vi "Get Transfer.vi"(10 "id":string, 11 "DSF Configuration in":T3) -> (0 "exists?":bool, 2 "info":T1, 3 "DSF Configuration out":T3, 4 "index":i32)   [LabVIEW 2017, in "DSF Core.lvlib" / "Configuration Session.lvclass"]
uses:
  Configuration Session.lvclass
  DSF Config Data.ctl
  Typedefs/DSF Timing Info.ctl
  DSF Core.lvlib
  Typedefs/DSF Version Info.ctl
  Internal DSF Configuration.ctl
  Typedefs/DSF Transfer Info.ctl
  Typedefs/DSF Byte Order.ctl
  Typedefs/DSF Settings Info.ctl
  Typedefs/DSF Engine Plugin Thread Configuration.ctl
  Typedefs/DSF File Format 1.0 Channel.ctl
  Typedefs/DSF File Format 1.0 Transfer.ctl
  Typedefs/DSF File Format 1.0 Transfer Group.ctl
  Typedefs/DSF File Format 1.0 Plugin.ctl
  Typedefs/DSF File Format 1.0 Framework v1.ctl
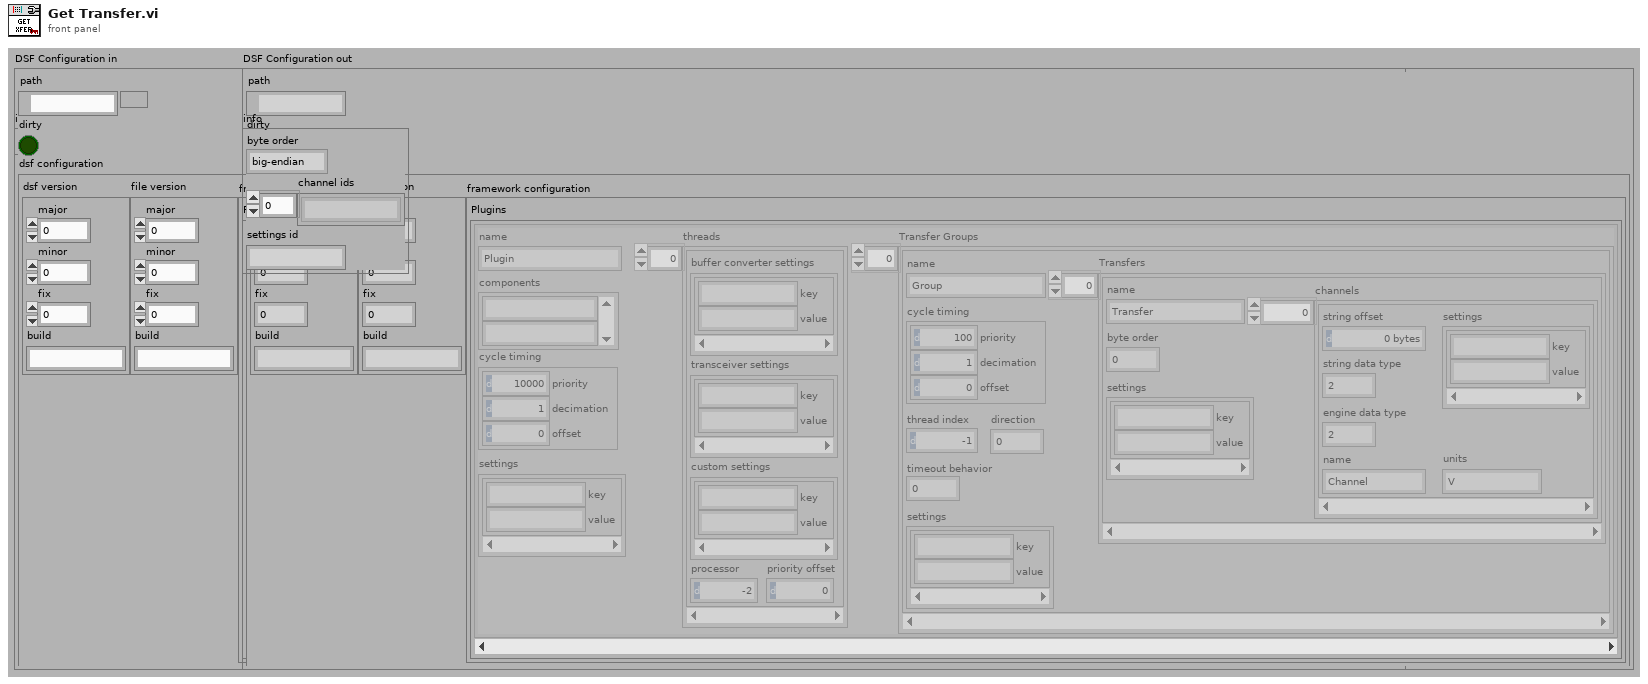
[diagram p1: front panel]
types:
  T1 = typedef "DSF Core.lvlib/DSF Transfer Info.ctl" = cluster{"byte order":T2, "channel ids":string[], "settings id":string}
  T2 = typedef "DSF Core.lvlib/DSF Byte Order.ctl" = enum8{"big-endian", "little-endian"}
  T3 = typedef "DSF Core.lvlib/Configuration Session.lvclass/DSF Config Data.ctl" = cluster{"path":path, "dirty":bool, "dsf configuration":T4}
  T4 = typedef "DSF Core.lvlib/Configuration Session.lvclass/Internal DSF Configuration.ctl" = cluster{"dsf version":T5, "file version":T5, "framework configuration":T6}
  T5 = typedef "DSF Core.lvlib/DSF Version Info.ctl" = cluster{"major":u32, "minor":u32, "fix":u32, "build":string}
  T6 = typedef "DSF Core.lvlib/Configuration Session.lvclass/DSF File Format 1.0 Framework v1.ctl" = cluster{"Plugins":T7[]}
  T7 = typedef "DSF Core.lvlib/Configuration Session.lvclass/DSF File Format 1.0 Plugin.ctl" = cluster{"name":string, "components":string[], "cycle timing":T8, "threads":T9[], "Transfer Groups":T11[], "settings":T10}
  T8 = typedef "DSF Core.lvlib/DSF Timing Info.ctl" = cluster{"priority":u64, "decimation":u64, "offset":u64}
  T9 = typedef "DSF Core.lvlib/DSF Engine Plugin Thread Configuration.ctl" = cluster{"buffer converter settings":T10, "transceiver settings":T10, "custom settings":T10, "processor":i32, "priority offset":i16}
  T10 = typedef "DSF Core.lvlib/DSF Settings Info.ctl" = cluster{"key":string, "value":string}[]
  T11 = typedef "DSF Core.lvlib/Configuration Session.lvclass/DSF File Format 1.0 Transfer Group.ctl" = cluster{"name":string, "direction":u8, "cycle timing":T8, "thread index":i32, "settings":T10, "Transfers":T12[], "timeout behavior":u8}
  T12 = typedef "DSF Core.lvlib/Configuration Session.lvclass/DSF File Format 1.0 Transfer.ctl" = cluster{"name":string, "byte order":u8, "settings":T10, "channels":T13[]}
  T13 = typedef "DSF Core.lvlib/Configuration Session.lvclass/DSF File Format 1.0 Channel.ctl" = cluster{"string offset":u64, "string data type":u8, "engine data type":u8, "name":string, "settings":T10, "units":string}
  T14 = typedef "DSF Core.lvlib/Configuration Session.lvclass/Internal DSF Transfer with ID.ctl" = cluster{"id":string, "values":T15}
  T15 = typedef "DSF Core.lvlib/Configuration Session.lvclass/Internal DSF Transfer Info.ctl" = cluster{"byte order":i32, "channel ids":string[], "settings id":string}
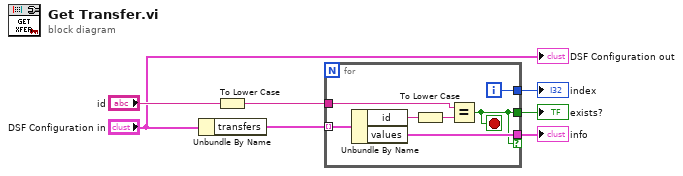
[diagram p0: block diagram]
diagram:
  n1 = Unbundle By Name("DSF Configuration in") -> ("transfers"=w7:T14[])
  n2 = To Lower Case(string="id") -> (all lower case string=w6:string)
  n3 = for {
    tunnel: w7 -> [w14] mode=indexing
    tunnel: w6 -> [w11]
    tunnel: [w8] -> w1
    tunnel: [w10] -> w2
    tunnel: [w9] -> w3 if=w8
    i -> [w10]
    stop <- w8 stop-if-true
    n4 = Unbundle By Name(w14) -> ("id"=w12:string, "values"=w9:T15)
    n5 = To Lower Case(string=w12) -> (all lower case string=w13:string)
    n6 = Equal?(x=w11, y=w13) -> (x = y?=w8:bool)
  }
  "index" <- w2
  "exists?" <- w1
  "info" <- w3
  "DSF Configuration out" <- "DSF Configuration in"
